vi "uObserver_Determine_Broker.vi"(8 "error in (no error)":errorcluster, 11 "uObserver in":refnum<class "uObserver.lvclass">) -> (0 "error out":errorcluster, 3 "uObserver out":refnum<class "uObserver.lvclass">)   [LabVIEW 2021, in "uFramework_pack_uActor.lvlib" / "uObserver.lvclass"]
doc: "Automatically checks upon initialization for a broker:\na) If it is a root actor, launch a new broker.\nb) If it is a nested actor, register to the broker available at the caller.\nc) Exception: If an actor reference is passed in using the accessor method prior to launching the actor, the actor ignores the caller's broker.\n\nA child override of this method may allow changing the abovementioned behavior. But in this case, the 'IsOwner?' flag must be set appropriately to prevent malfunctional behavior on actor's shutdown.\n\n<B>This is called before the uActor's Init method.</B> On error, the observer actor will fail to launch and will not invoke the uActor ErrHandling method. It will just return a nested-actor-stop message to the caller."
uses:
  uObserver.lvclass
  uObserver.lvclass/uObserver.ctl
  Bin/uFramework.lvlibp/uTransport_uActor/uTransport_uActor.lvclass
  U:/Projects/uFramework/Bin/uFramework.lvlibp/uTransport/uTransport.lvclass
  Bin/uFramework.lvlibp/uBroker/uBroker.lvclass
  Bin/uData.lvlibp/uData.lvclass
  Bin/uFramework.lvlibp/uActor/uActor.lvclass
  Bin/uFramework.lvlibp/uTransport/uTransport.lvclass
  U:/Projects/uFramework/Bin/uFramework.lvlibp/uActor/uActor.lvclass
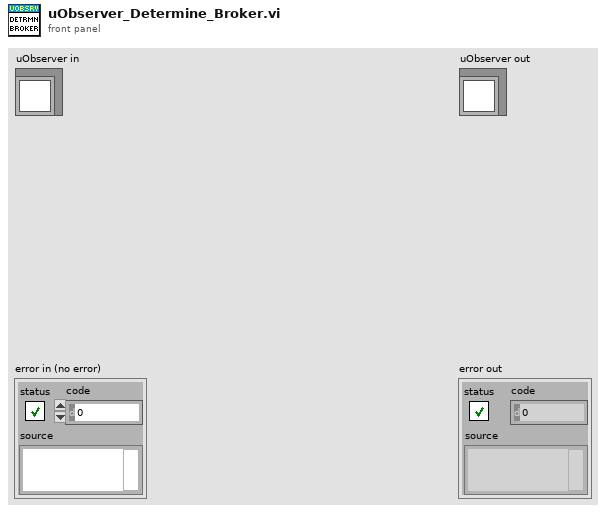
[diagram p1: front panel]
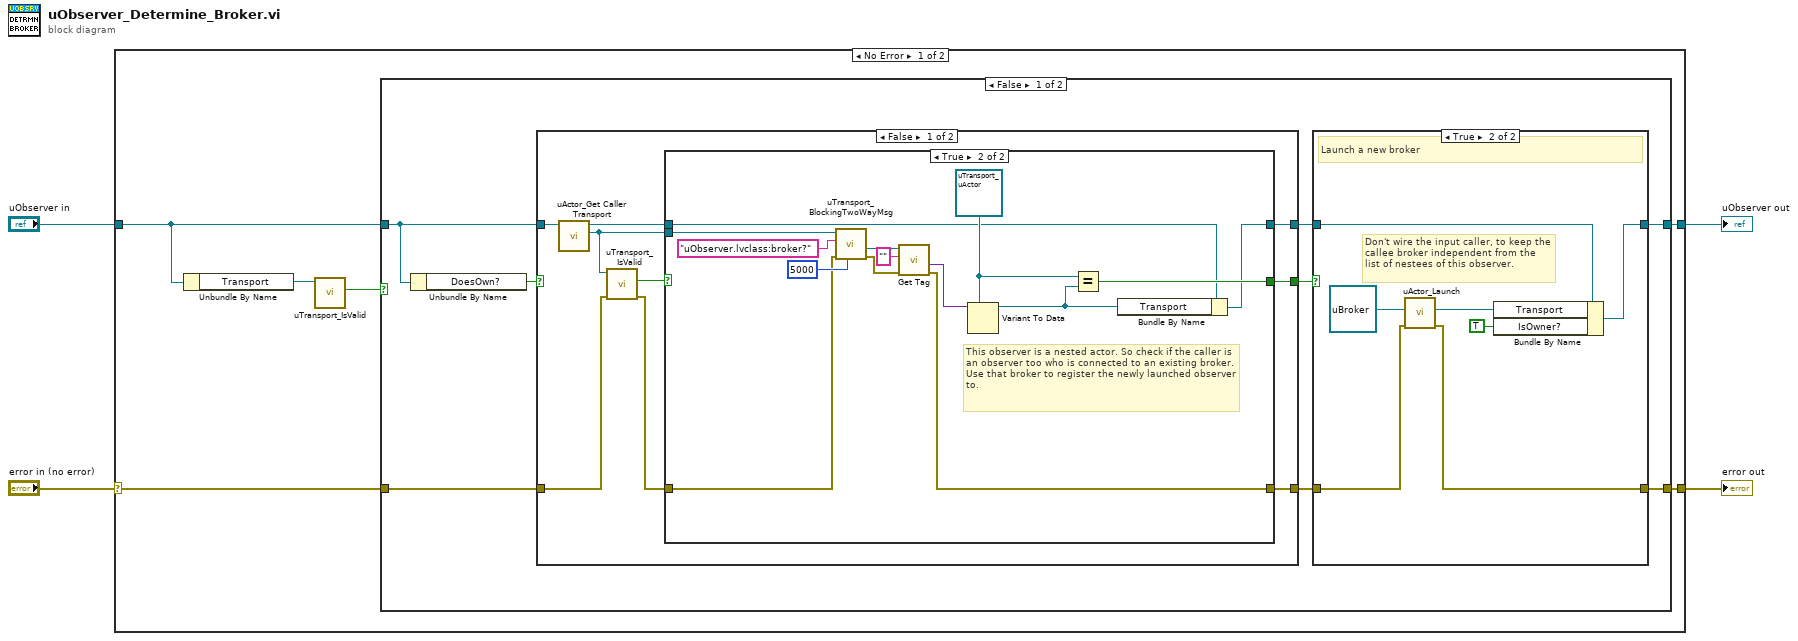
[diagram p0: block diagram]
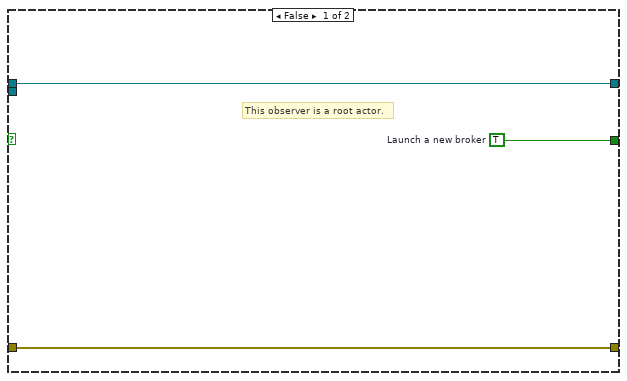
[diagram p2: hidden frame]
diagram:
  n1 = case shown="No Error" "error in (no error)" {
    selector: "error in (no error)" -> [w6 w60]
    tunnel: [w5 w60] -> w3
    tunnel: [w7 w59] -> w1
    tunnel: "uObserver in" -> [w8 w59]
    frame No Error {
      n2 = Unbundle By Name(w8) -> ("Transport"=w10:refnum<class "uTransport_uActor.lvclass">)
      n3 = call-dynamic "uTransport_IsValid.vi"("uTransport_uActor in"=w10) -> ("IsValid?"=w9:bool)  [unwired: 8 in, 2 out]
      n4 = case shown="False" w9 {
        tunnel: w8 -> [w12 w58]
        tunnel: [w15 w58] -> w7
        tunnel: w6 -> [w18 w57]
        tunnel: [w13 w57] -> w5
        frame False {
          n5 = Unbundle By Name(w12) -> ("DoesOwn?"=w11:bool)
          n6 = case shown="False" w11 {
            selector: w11 -> [_ w47]
            tunnel: w18 -> [w25 w45]
            tunnel: [w23 w46] -> w17
            tunnel: [w22 w47] -> w16
            tunnel: [w21 w45] -> w14
            tunnel: w12 -> [w20 w46]
            frame False {
              n7 = call "uActor_Get Caller Transport.vi"("uActor in"=w20) -> ("Caller's Transport"=w19:refnum<class "uTransport_uActor.lvclass">, "uActor out"=w24:refnum<class "uObserver.lvclass">)  [unwired: 9 in]
              n8 = call-dynamic "uTransport_IsValid.vi"("error in (no error)"=w25, "uTransport_uActor in"=w19) -> ("error out"=w26:errorcluster, "IsValid?"=w27:bool)  [unwired: 7 in, 1 out]
              n9 = case shown="True" w27 {
                tunnel: w26 -> [w29 w37]
                tunnel: [w29 w38] -> w21
                tunnel: w24 -> [w30 w32]
                tunnel: [w30 w33] -> w23
                tunnel: [w28 w34] -> w22
                tunnel: w19 -> [_ w44]
                frame False {
                  w28 = TRUE  # Launch a new broker
                  # "This observer is a root actor."
                }
                frame True {
                  w35 = refnum<class "uTransport_uActor.lvclass"> refnum ("uFramework.lvlibp:uTransport_uActor.lvclass")
                  # "This observer is a nested actor. So check if the caller is an observer too who is connected to an existing broker. Use that broker to register the newly launched observer to."
                  n10 = call "uTransport_BlockingTwoWayMsg.vi"("timeout in ms (5000)"=5000, "error in (no error)"=w37, "Command"="uObserver.lvclass:broker?", "uActor Transport"=w44) -> ("error out"=w41:errorcluster, "Reply"=w43:refnum<class "uData.lvclass">)  [unwired: 6 in]
                  n11 = call "Get Tag.vi"("error in (no error)"=w41, "tag (case insensitive)"="", "uData in"=w43) -> ("error out"=w38:errorcluster, "value"=w36:variant)  [unwired: 5 in, 2 out]
                  n12 = Variant To Data(type=w35, Variant=w36) -> (data=w31:refnum<class "uTransport_uActor.lvclass">)  [unwired: 1 in, 1 out]
                  n13 = Equal?(x=w35, y=w31) -> (x = y?=w34:bool)
                  n14 = Bundle By Name(cluster=w32, "Transport"=w31) -> (w33:refnum<class "uObserver.lvclass">)
                }
              }
            }
            frame True {
            }
          }
          n15 = case shown="True" w16 {
            tunnel: w14 -> [w48 w54]
            tunnel: [w48 w55] -> w13
            tunnel: w17 -> [w49 w52]
            tunnel: [w49 w53] -> w15
            frame False {
              # "Don't create a new broker"
            }
            frame True {
              # "Don't wire the input caller, to keep the callee broker independent from the list of nestees of this observer."
              # "Launch a new broker"
              n16 = call "uActor_Launch.vi"("error in (no error)"=w54, "Actor to Launch"=refnum<class "uBroker.lvclass"> refnum ("uFramework.lvlibp:uBroker.lvclass")) -> ("error out"=w55:errorcluster, "uTransport_uActor"=w51:refnum<class "uTransport_uActor.lvclass">)  [unwired: 7 in, 1 out]
              n17 = Bundle By Name(cluster=w52, "Transport"=w51, "IsOwner?"=TRUE ("Broker.IsOwner?")) -> (w53:refnum<class "uObserver.lvclass">)
            }
          }
        }
        frame True {
          # "A broker's reference has been passed in using the accessor method prior to calling this VI. This supersedes everything else. No Broker actor is created and the caller's broker is not used for this newly launched observer."
        }
      }
    }
    frame Error {
    }
  }
  "error out" <- w3
  "uObserver out" <- w1
